vi "outdoor_temp.vi"(1 "temp max":dbl, 2 "temp min":dbl, 3 "time in":dbl) -> (0 "temp out":dbl)   [LabVIEW 2014]
uses:
  <vilib>/Analysis/1siggen.llb/Ramp Pattern by Samples.vi
  <vilib>/Analysis/NI_AALBase.lvlib
panel:
  out "XY Graph":T1(graph)
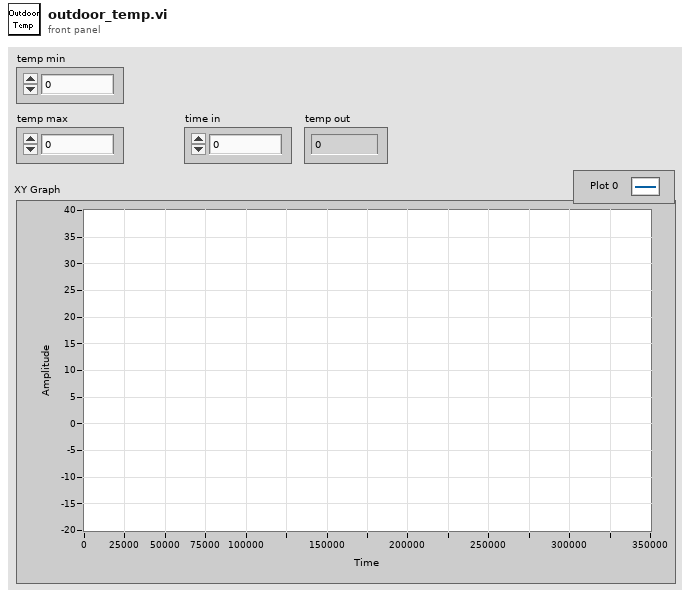
[diagram p1: front panel]
types:
  T1 = cluster{"Ramp Pattern":dbl[], "Ramp Pattern":dbl[]}
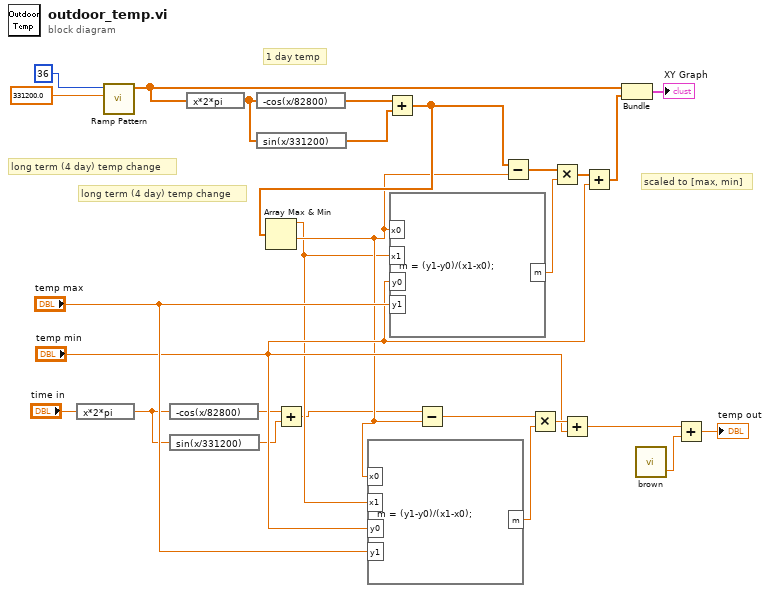
[diagram p0: block diagram]
diagram:
  # "long term (4 day) temp change"
  # "scaled to [max, min]"
  # "1 day temp"
  # "long term (4 day) temp change"
  n1 = expression code="x*2*pi"("time in") -> (w1:dbl)
  n2 = call-poly <vilib>:"Ramp Pattern.vi"("end"=331200.0 ("end hour"), "samples"=36) -> ("Ramp Pattern"=w20:dbl[])  [unwired: 8 in, 1 out]
  n3 = expression code="-cos(x/82800)"(w1) -> (w4:dbl)
  n4 = expression code="sin(x/331200)"(w1) -> (w3:dbl)
  n5 = expression code="x*2*pi"(w20) -> (w9:dbl[])
  n6 = expression code="-cos(x/82800)"(w9) -> (w11:dbl[])
  n7 = expression code="sin(x/331200)"(w9) -> (w10:dbl[])
  n8 = Add(x=w4, y=w3) -> (x+y=w2:dbl)
  n9 = Add(x=w11, y=w10) -> (x+y=w8:dbl[])
  n10 = Array Max & Min(array=w8) -> (max value=w5:dbl, min value=w6:dbl)  [unwired: 2 out]
  n11 = formula code="m = (y1-y0)/(x1-x0);"("x0"=w6, "x1"=w5, "y0"="temp min", "y1"="temp max") -> ("m"=w18:dbl)
  n12 = formula code="m = (y1-y0)/(x1-x0);"("x0"=w6, "x1"=w5, "y0"="temp min", "y1"="temp max") -> ("m"=w24:dbl)
  n13 = Subtract(x=w2, y=w6) -> (x-y=w17:dbl)
  n14 = Subtract(x=w8, y=w6) -> (x-y=w25:dbl[])
  n15 = Multiply(x=w17, y=w18) -> (x*y=w19:dbl)
  n16 = Multiply(x=w25, y=w24) -> (x*y=w22:dbl[])
  n17 = Add(x=w19, y="temp min") -> (x+y=w12:dbl)
  n18 = Add(x=w22, y="temp min") -> (x+y=w21:dbl[])
  n19 = Bundle("Ramp Pattern"=w20, w21) -> (→"XY Graph":cluster{"Ramp Pattern":dbl[], dbl[]})  [unwired: 1 in]
  n20 = call "brown.vi"() -> ("brown/2"=w7:dbl)  [unwired: 1 in, 1 out]
  n21 = Add(x=w12, y=w7) -> (x+y=→"temp out":dbl)
